vi "Estimate Substitution.vi"(8 "error in (no error)":errorcluster, 11 "Vessel in":refnum<class "Vessel.lvclass">) -> (0 "error out":errorcluster, 3 "Vessel out":refnum<class "Vessel.lvclass">)   [LabVIEW 2014, in "Vessel.lvclass"]
uses:
  Vessel.lvclass
  Vessel.lvclass/Vessel.ctl
  Supervisor/Supervisor.lvclass
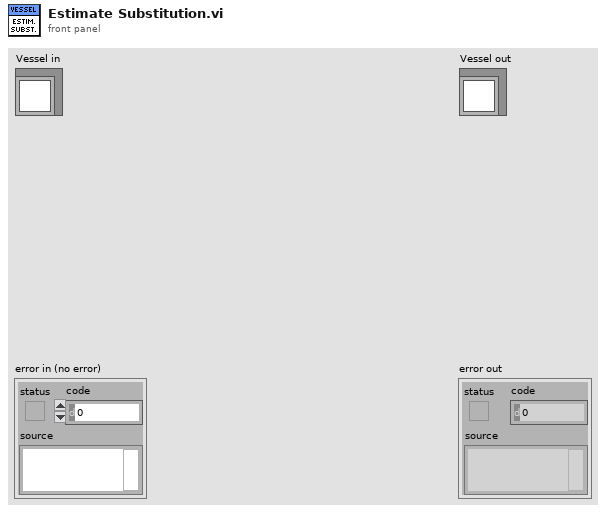
[diagram p1: front panel]
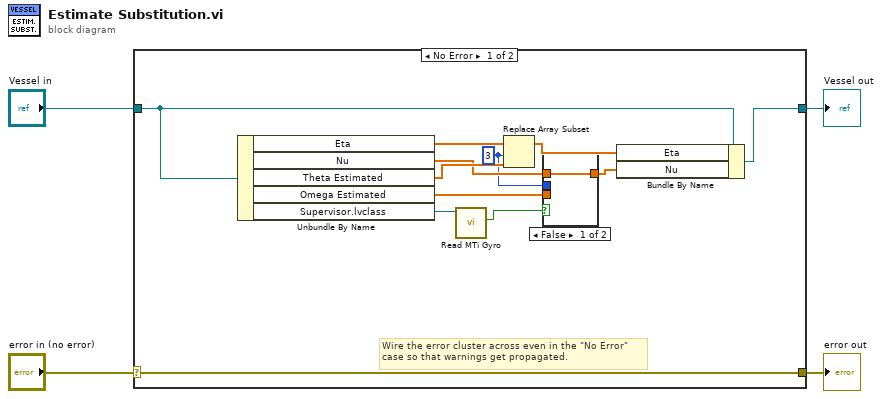
[diagram p0: block diagram]
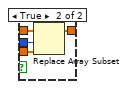
[diagram p2: hidden frame]
diagram:
  n1 = case shown="No Error" "error in (no error)" {
    selector: "error in (no error)" -> [w16 w23]
    tunnel: [w16 w23] -> w3
    tunnel: [w9 w22] -> w1
    tunnel: "Vessel in" -> [w10 w22]
    frame No Error {
      w11 = 3 ("index")
      # "Wire the error cluster across even in the \"No Error\"\ncase so that warnings get propagated."
      n2 = Unbundle By Name(w10) -> ("Eta"=w15:dbl[], "Nu"=w13:dbl[], "Theta Estimated"=w14:dbl[], "Omega Estimated"=w12:dbl[], "Supervisor.lvclass"=w6:refnum<class "Supervisor.lvclass">)
      n3 = call-dynamic "Read MTi Gyro.vi"("Supervisor in"=w6) -> ("MTi Gyro"=w5:bool)  [unwired: 8 in, 2 out]
      n4 = Replace Array Subset(array=w15, new element=w14, index=w11) -> (w8:dbl[])
      n5 = case shown="False" w5 {
        tunnel: w13 -> [w17 w21]
        tunnel: w12 -> [_ w20]
        tunnel: w11 -> [_ w19]
        tunnel: [w17 w18] -> w7
        frame False {
        }
        frame True {
          n6 = Replace Array Subset(array=w21, new element=w20, index=w19) -> (w18:dbl[])
        }
      }
      n7 = Bundle By Name(cluster=w10, "Eta"=w8, "Nu"=w7) -> (w9:refnum<class "Vessel.lvclass">)
    }
    frame Error {
    }
  }
  "error out" <- w3
  "Vessel out" <- w1
